vi "Save CD XML.vi"(8 "error in (no error)":errorcluster, 11 "Project XML Editor in":refnum<class "Project XML Editor.lvclass">) -> (0 "error out":errorcluster, 3 "Project XML Editor out":refnum<class "Project XML Editor.lvclass">)   [LabVIEW 2020, in "LVLIBP CD XML Updater.lvlib" / "Project XML Editor.lvclass"]
uses:
  Project XML Editor.lvclass
  Project XML Editor.lvclass/Project XML Editor.ctl
  <resource>/objmgr/DOMUserDefRef.rc
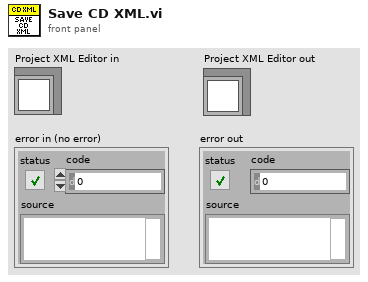
[diagram p1: front panel]
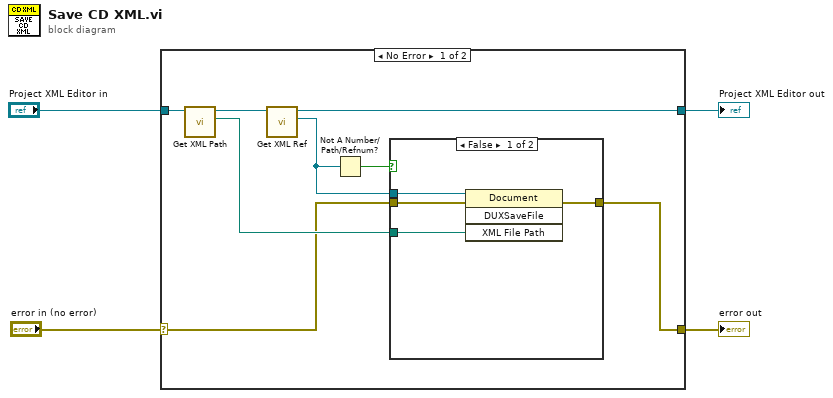
[diagram p0: block diagram]
diagram:
  n1 = case shown="No Error" "error in (no error)" {
    selector: "error in (no error)" -> [w5 w19]
    tunnel: [w12 w19] -> w4
    tunnel: "Project XML Editor in" -> [w9 w18]
    tunnel: [w6 w18] -> w2
    frame No Error {
      n2 = call "Get XML Path.vi"("Project XML Editor in"=w9) -> ("XML Path"=w11:path, "Project XML Editor out"=w10:refnum<class "Project XML Editor.lvclass">)  [unwired: 9 in]
      n3 = call "Get XML Ref.vi"("Project XML Editor in"=w10) -> ("XML Ref"=w8:refnum<k20>, "Project XML Editor out"=w6:refnum<class "Project XML Editor.lvclass">)  [unwired: 9 in]
      n4 = Not A Number/Path/Refnum?(number/path/refnum=w8) -> (NaN/Path/Refnum?=w7:bool)
      n5 = case shown="False" w7 {
        tunnel: w8 -> [w16 _]
        tunnel: w11 -> [w15 _]
        tunnel: w5 -> [w14 w17]
        tunnel: [w13 w17] -> w12
        frame False {
          n6 = invoke class="Document" method="DUXSaveFile"(reference=w16, error in=w14, "XML File Path"=w15) -> (error out=w13:errorcluster)  [unwired: 1 in, 3 out]
        }
        frame True {
        }
      }
    }
    frame Error {
    }
  }
  "error out" <- w4
  "Project XML Editor out" <- w2
